vi "PWMTest.vi"() -> ()   [LabVIEW 2009]
uses:
  PWM/PWM_Name.ctl
  <vilib>/Platform/TimedLoop/XDataNode/XDataNode.xnode
  <vilib>/Platform/TimedLoop/XDataNode/loadlvalarms.vi
  <vilib>/Platform/TimedLoop/XDataNode/timing_clust.ctl
  <vilib>/Platform/TimedLoop/XDataNode/nitl_modes.ctl
  <vilib>/Platform/TimedLoop/XDataNode/wakeup.ctl
  <vilib>/Platform/TimedLoop/XDataNode/XDNodeRunTimeDep.lvlib
  PWM.lvlib
  FPGA.lvlib
panel:
  in  "PWM":T1=9 items=["Invalid"=0, "PWM1"=1, "PWM2"=2, "PWM9"=9, "PWM10"=10]
  in  "PWM1_Enable":bool
  in  "PWM1":cluster{"High (uSec)":u32, "Period (uSec)":u32} {"High (uSec)" scale=900.0..2100.0}
  in  "PWM10_Enable":bool
  in  "PWM9_Enable":bool
  in  "PWM10":cluster{"High (uSec)":u32, "Period (uSec)":u32}={"High (uSec)"=1360, "Period (uSec)"=0} {"High (uSec)" min=1360 max=2200 scale=1360.0..2200.0}
  in  "PWM9":cluster{"High (uSec)":u32, "Period (uSec)":u32}={"High (uSec)"=930, "Period (uSec)"=0} {"High (uSec)" min=930 max=1770 scale=930.0..1770.0}
  in  "stop":bool
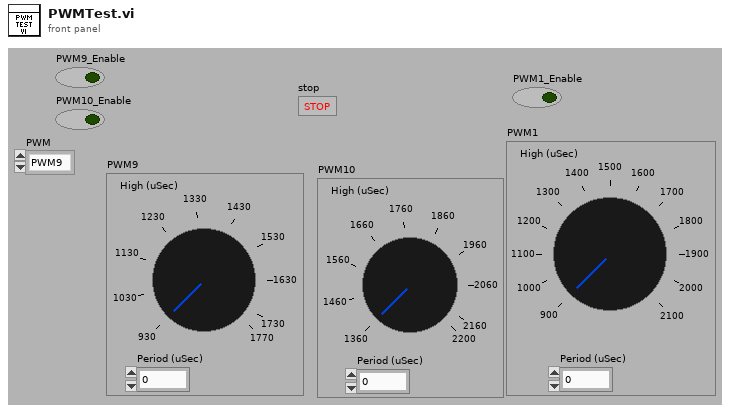
[diagram p1: front panel]
types:
  T1 = typedef "PWM.lvlib/PWM_Name.ctl" = u16
  T2 = typedef "XDNodeRunTimeDep.lvlib/timing_clust.ctl" = cluster{"Expected End [f-1]":u64, "Actual End [f-1]":u64, "Finished Late? [f-1]":bool, "Expected End [i-1]":u64, "Actual End [i-1]":u64, "Finished Late? [i-1]":bool, "Expected Start [i]":u64, "Actual Start [i]":u64, "Expected Start [f]":u64, "Actual Start [f]":u64, "Source Name":string, "Structure Name":string, "Period":i64, "Deadline":i64, "Offset":i64, "Start":i64, "Priority":i32, "Timeout":i32, "Mode":T3, "Wakeup Reason":T4, "Error":errorcluster, "Source Type":string, "Secondary Source Type":string, "Global End Time":u64, "Global Start Time":u64, "Frame Duration":u64, "Iteration Duration":u64, "Assigned CPU":i32, "I/O Scan Engine Mode":u32}
  T3 = typedef "XDNodeRunTimeDep.lvlib/nitl_modes.ctl" = enum32{"No Change", "Process missed periods, maintain original phase", "Discard missed periods, maintain original phase", "Process missed periods, ignore original phase", "Discard missed periods, ignore original phase"}
  T4 = typedef "XDNodeRunTimeDep.lvlib/wakeup.ctl" = enum32{"Normal", "Aborted", "Asynchronous wakeup", "Timing source error", "Timed loop error", "Timeout"}
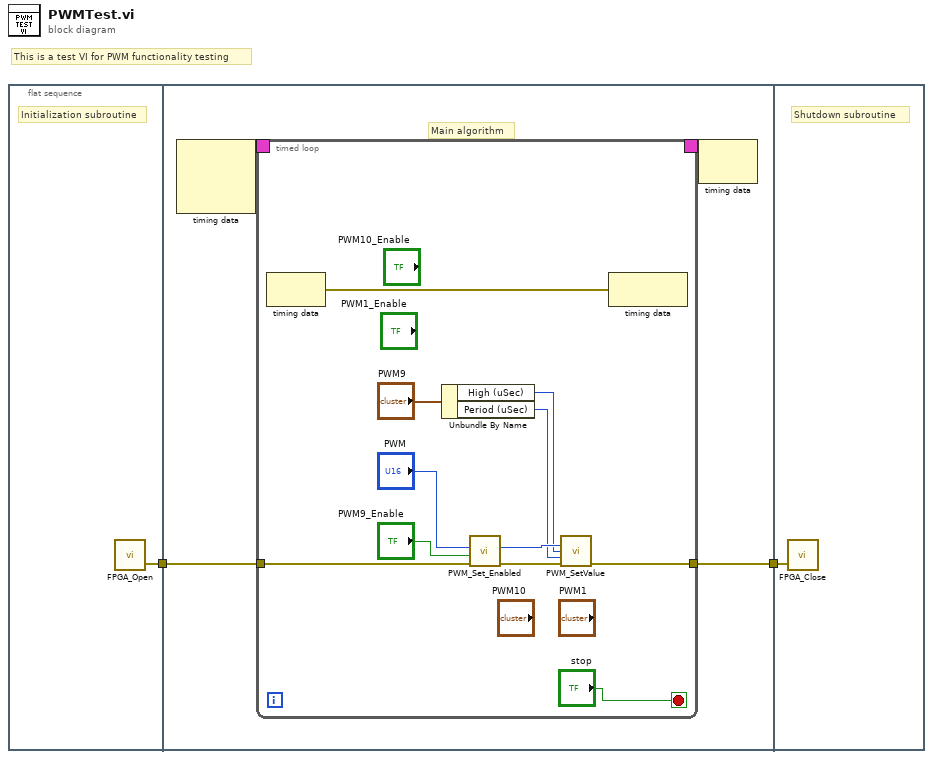
[diagram p0: block diagram]
diagram:
  # "This is a test VI for PWM functionality testing"
  n1 = flat-sequence {
    tunnel: [w3] -> w2
    tunnel: w2 -> [w5]
    tunnel: [w4] -> w1
    tunnel: w1 -> [w26]
    frame #0 {
      # "Initialization subroutine"
      n2 = call "FPGA_Open.vi"() -> ("error out"=w3:errorcluster)  [unwired: 3 in]
    }
    frame #1 {
      # "Main algorithm"
      n3 = node-c288() -> (w7:T2)  [unwired: 3 in]
      n4 = timed-loop {
        timing: w7 -> [_]
        timing-out: [_] -> w6
        tunnel: w5 -> [w8]
        tunnel: [w14] -> w4
        stop <- "stop" stop-if-true
        n5 = node-c288() -> (w17:errorcluster)  [unwired: 1 in]
        n6 = Unbundle By Name("PWM9") -> ("High (uSec)"=w10:u32, "Period (uSec)"=w9:u32)
        n7 = call "PWM_Set_Enabled.vi"("error in"=w8, "Enable"="PWM9_Enable", "PWM_in"="PWM") -> ("error out"=w13:errorcluster, "PWM_out"=w12:T1)  [unwired: 7 in]
        n8 = call "PWM_SetValue.vi"("PWM"=w12, "High (uSec)"=w10, "Period (uSec)"=w9, "error in"=w13) -> ("error out"=w14:errorcluster)  [unwired: 11 in]
        n9 = node-c288(w17) -> ()  [unwired: 1 out]
      }
      n10 = node-c288(w6) -> ()  [unwired: 1 out]
    }
    frame #2 {
      # "Shutdown subroutine"
      n11 = call "FPGA_Close.vi"("error in (no error)"=w26) -> ()  [unwired: 2 in, 1 out]
    }
  }
